vi "pressure_report.vi"(8 "Error In":errorcluster, 11 "Pressure data":T1) -> (0 "Error Out":errorcluster)   [LabVIEW 2016]
uses:
  pressure_data.ctl
  Report/report_mods.ctl
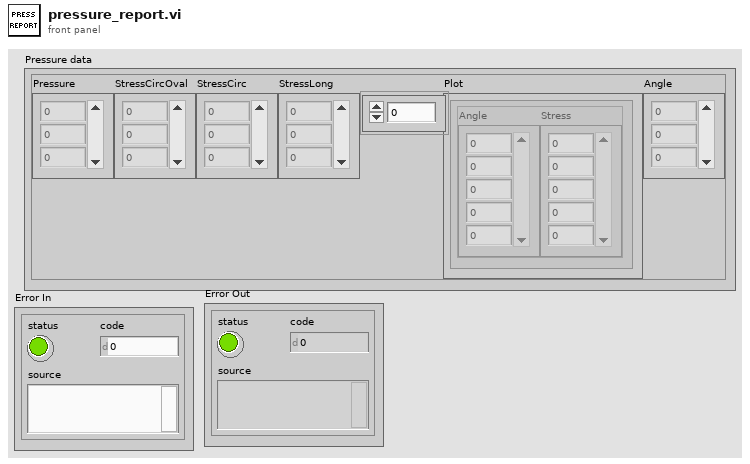
[diagram p1: front panel]
types:
  T1 = typedef "pressure_data.ctl" = cluster{"Pressure":dbl[], "StressCircOval":dbl[], "StressCirc":dbl[], "StressLong":dbl[], "Plot":cluster{"Angle":dbl[], "Stress":dbl[]}[], "Angle":dbl[]}
  T2 = typedef "report_mods.ctl" = enum16{"Init", "Table", "Graph", "TablefromGraph", "End"}
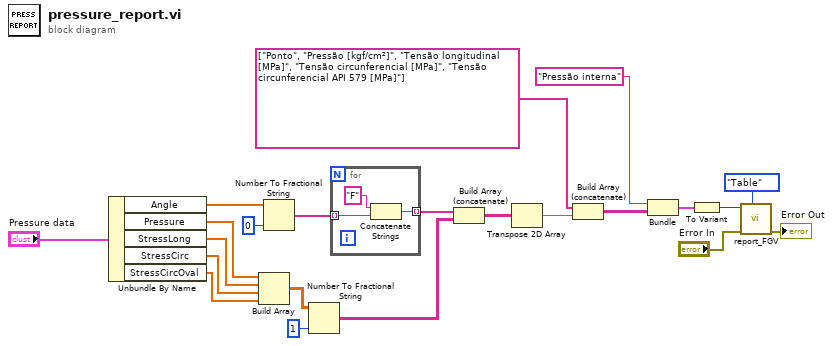
[diagram p0: block diagram]
diagram:
  n1 = Unbundle By Name("Pressure data") -> ("Angle"=w21:dbl[], "Pressure"=w18:dbl[], "StressLong"=w17:dbl[], "StressCirc"=w16:dbl[], "StressCircOval"=w15:dbl[])
  n2 = Build Array(w18, w17, w16, w15) -> (w13:dbl[][])
  n3 = Number To Fractional String(number=w21, precision (6)=i16 0) -> (F-format string=w19:string[])  [unwired: 2 in]
  n4 = Number To Fractional String(number=w13, precision (6)=i16 1) -> (F-format string=w11:string[][])  [unwired: 2 in]
  n5 = for {
    tunnel: w19 -> [w25] mode=indexing
    tunnel: [w23] -> w12 mode=indexing
    n6 = Concatenate Strings("F" ("string"), w25) -> (w23:string)
  }
  n7 = Build Array (concatenate)(w12, w11) -> (w10:string[][])
  n8 = Transpose 2D Array(2D array=w10) -> (transposed array=w9:string[][])
  n9 = Build Array (concatenate)(string[] ["Ponto", "Pressão [kgf/cm²]", "Tensão longitudinal [MPa]", "Tensão circunferencial [MPa]", "Tensão circunferencial API 579 [MPa]"] ("element"), w9) -> (w7:string[][])
  n10 = Bundle("Numeric"="Pressão interna", w7) -> (w5:cluster{"Numeric":string, string[][]})  [unwired: 1 in]
  n11 = To Variant(anything=w5) -> (Variant=w4:variant)
  n12 = call "report_FGV.vi"("report_mods"=report_mods."Table", "Error In"="Error In", "Data in"=w4) -> ("Error Out"=→"Error Out":errorcluster)  [unwired: 8 in]
